vi "Write Sub Panel Coin.vi"(8 "error in (no error)":errorcluster, 10 "Sub Panel Coin":refnum<vi>, 11 "Monedas MXN in":refnum<class "Monedas MXN.lvclass">) -> (0 "error out":errorcluster, 3 "Monedas MXN out":refnum<class "Monedas MXN.lvclass">)   [LabVIEW 2020, in "Monedas MXN.lvlib" / "Monedas MXN.lvclass"]
uses:
  Monedas MXN.lvclass
  Monedas MXN.lvclass/Monedas MXN.ctl
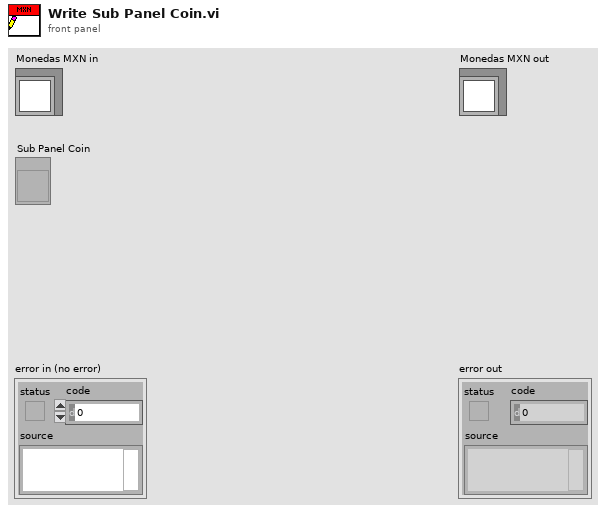
[diagram p1: front panel]
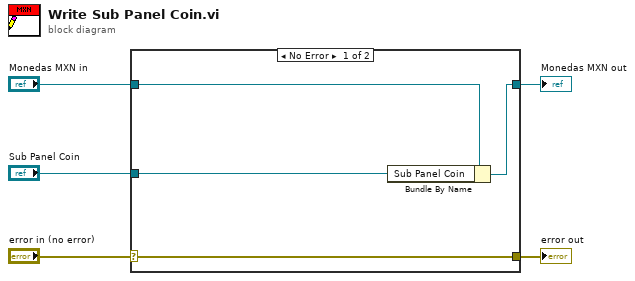
[diagram p0: block diagram]
diagram:
  n1 = case shown="No Error" "error in (no error)" {
    selector: "error in (no error)" -> [w9 w10]
    tunnel: [w9 w10] -> w4
    tunnel: [w7 w11] -> w2
    tunnel: "Monedas MXN in" -> [w8 w11]
    tunnel: "Sub Panel Coin" -> [w6 _]
    frame No Error {
      n2 = Bundle By Name(cluster=w8, "Sub Panel Coin"=w6) -> (w7:refnum<class "Monedas MXN.lvclass">)
    }
    frame Error {
    }
  }
  "error out" <- w4
  "Monedas MXN out" <- w2
